vi "New.vi"(8 "error in (no error)":errorcluster, 10 "Secret":string) -> (0 "error out":errorcluster, 3 "output cluster":refnum<class "WampCraAuthenticator.lvclass">)   [LabVIEW 2020, in "wamplv.lvlib" / "WampCraAuthenticator.lvclass"]
uses:
  WampCraAuthenticator.lvclass
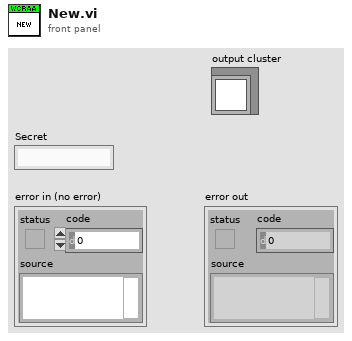
[diagram p1: front panel]
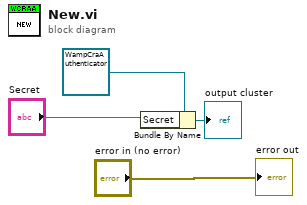
[diagram p0: block diagram]
diagram:
  n1 = Bundle By Name(cluster=refnum<class "WampCraAuthenticator.lvclass"> refnum ("wamplv.lvlib:WampCraaAuthenticator.lvclass"), "Secret"="Secret") -> (→"output cluster":refnum<class "WampCraAuthenticator.lvclass">)
  "error out" <- "error in (no error)"
